vi "New image.vi"(8 "error in (no error)":errorcluster, 9 "Buffer Number":u32, 10 "Image":T1, 11 "Camera Tester in":refnum<class "Camera Tester.lvclass">) -> (0 "error out":errorcluster, 3 "Camera Tester out":refnum<class "Camera Tester.lvclass">)   [LabVIEW 2014, in "Camera Tester.lvlib" / "Camera Tester.lvclass"]
uses:
  Camera Tester.lvclass
  <vilib>/vision/Image Controls.llb/IMAQ Image.ctl
  Camera Tester.lvclass/Camera Tester.ctl
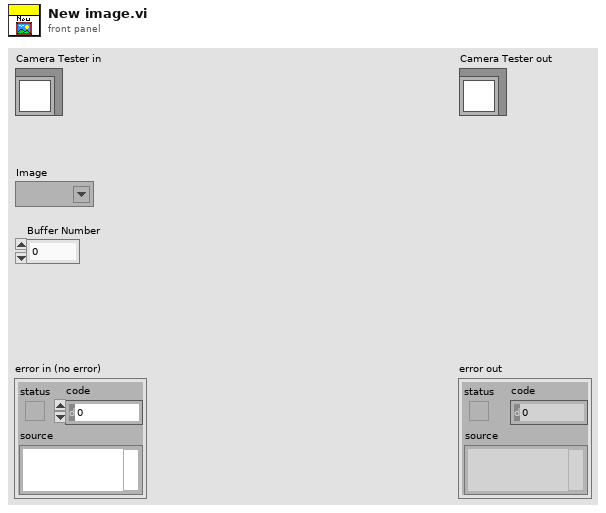
[diagram p1: front panel]
types:
  T1 = typedef "IMAQ Image.ctl" = refnum<image>
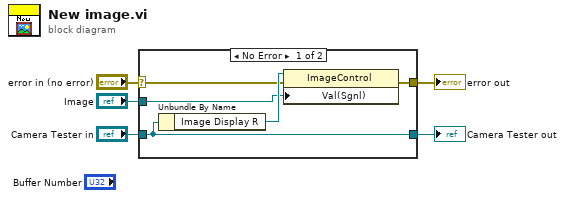
[diagram p0: block diagram]
diagram:
  n1 = case shown="No Error" "error in (no error)" {
    selector: "error in (no error)" -> [w7 w12]
    tunnel: [w6 w12] -> w4
    tunnel: [w10 w11] -> w2
    tunnel: "Camera Tester in" -> [w10 w11]
    tunnel: "Image" -> [w8 _]
    frame No Error {
      n2 = Unbundle By Name(w10) -> ("Image Display R"=w9:refnum<vi>)
      n3 = property class="ImageControl"(reference=w9, error in=w7, "Val(Sgnl)"=w8) -> (error out=w6:errorcluster)  [unwired: 1 out]
    }
    frame Error {
    }
  }
  "error out" <- w4
  "Camera Tester out" <- w2
